vi "MQTT_TCP_Close_Connection.vi"(8 "error in (no error)":errorcluster, 10 "abort (F)":bool, 11 "connection ID":refnum<k5>) -> (0 "error out":errorcluster, 3 "connection ID out":refnum<k5>)   [LabVIEW 2017, in "MQTT_Functions.lvlib"]
uses:
  MQTT_Functions.lvlib
panel:
  # "this is just a wrapper for the TCP Close Connection function\nadd or replace functionality as desired"
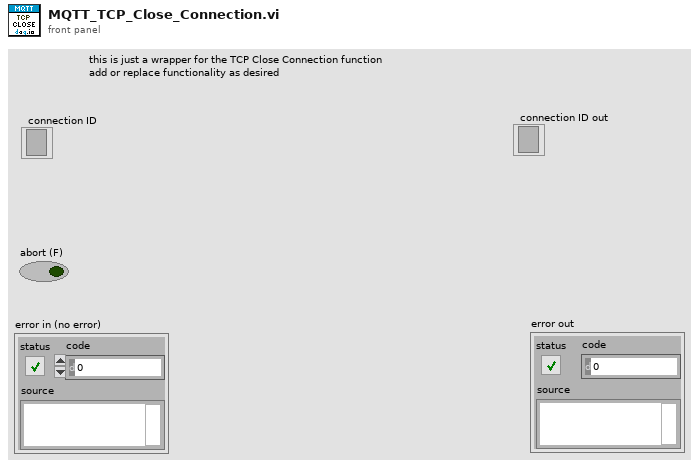
[diagram p1: front panel]
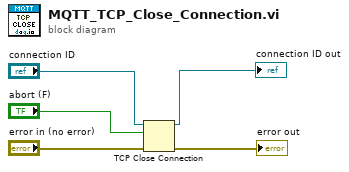
[diagram p0: block diagram]
diagram:
  n1 = TCP Close Connection(connection ID="connection ID", abort (F)="abort (F)", error in (no error)="error in (no error)") -> (connection ID out=→"connection ID out":refnum<k5>, error out=→"error out":errorcluster)
